vi "Global.vi"() -> ()   [LabVIEW 2011, in "Sensor Simulation Custom Device.lvlib"]
uses:
  Sensor Simulation Custom Device.lvlib
panel:
  in  "FPGA RT Path":string="FPGA RT Path"
  in  "Init Failed":string="Init Failed"
  in  "Main Page GUID_Disable":string="F11B1F54-08E1-5F2A-9C34-B780B7E96084"
  in  "Sensor Type":string="Sensor Type"
  in  "Resolver Setup":string="Resolver Setup"
  in  "Resolver Page":string="AA3C26FC-1E5E-48BF-EE97-8EBAE534A484"
  in  "xVDT TransRatio":string="xVDT TransRatio"
  in  "xVDT Sensitivity":string="xVDT Sensitivity"
  in  "xVDT Setup":string="xVDT Setup"
  in  "xVDT Page":string="B55E918E-A064-4774-772A-614E6E638C7C"
  in  "Main Page GUID_Enable":string="1EB611CB-5887-3E13-F70F-E119B75BBCCF"
  in  "Channel Del Prot GUID":string="1F74E8F6-DA20-CAEC-33C8-172BA5430576"
  in  "FPGA Type":string="FPGA Type"
  in  "FPGA Path":string="FPGA Path"
  in  "FPGA Checksum":string="FPGA Checksum"
  in  "FPGA Name":string="FPGA Name"
  in  "FPGA Reference":string="FPGA Reference"
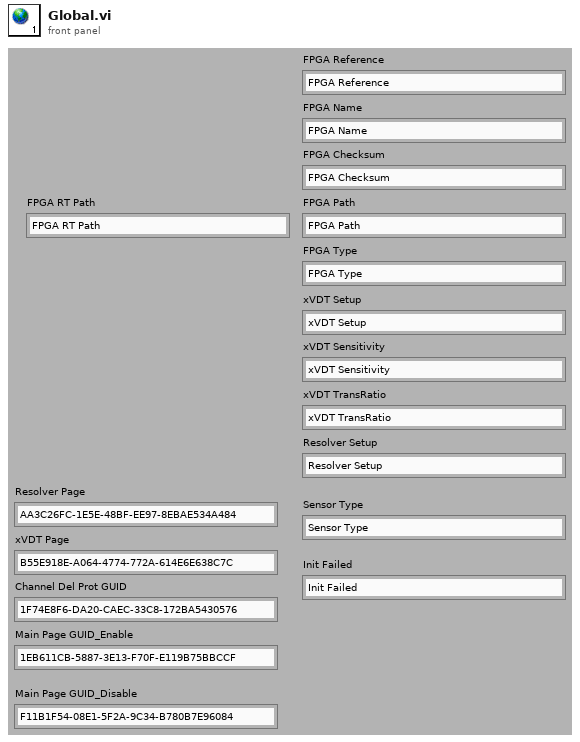
[diagram p1: front panel]
diagram:
